vi "Pasco Drive Correcting.vi"(11 "Power":dbl) -> (0 "RightDriveOutput":dbl, 3 "LeftDriveOutput":dbl)   [LabVIEW 2011]
uses:
  Robot Global Data.vi
panel:
  in  "LeftDriveOutput 2":dbl
  in  "RightDriveOutput 2":dbl
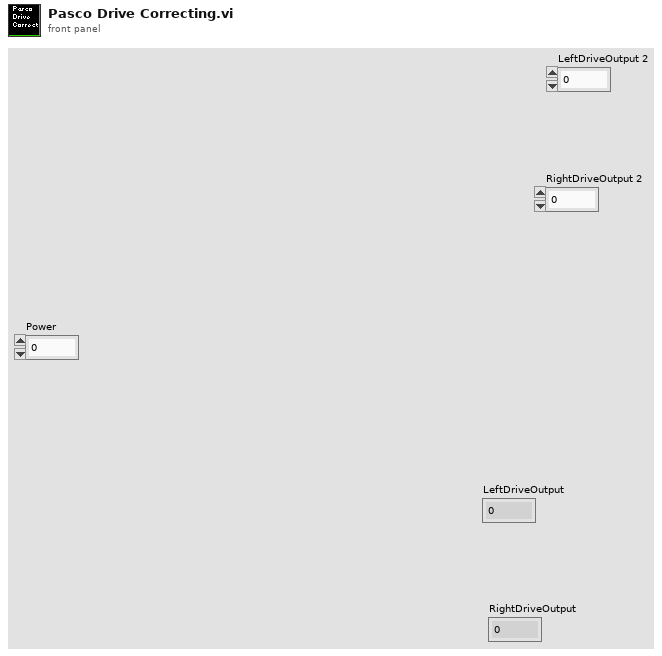
[diagram p1: front panel]
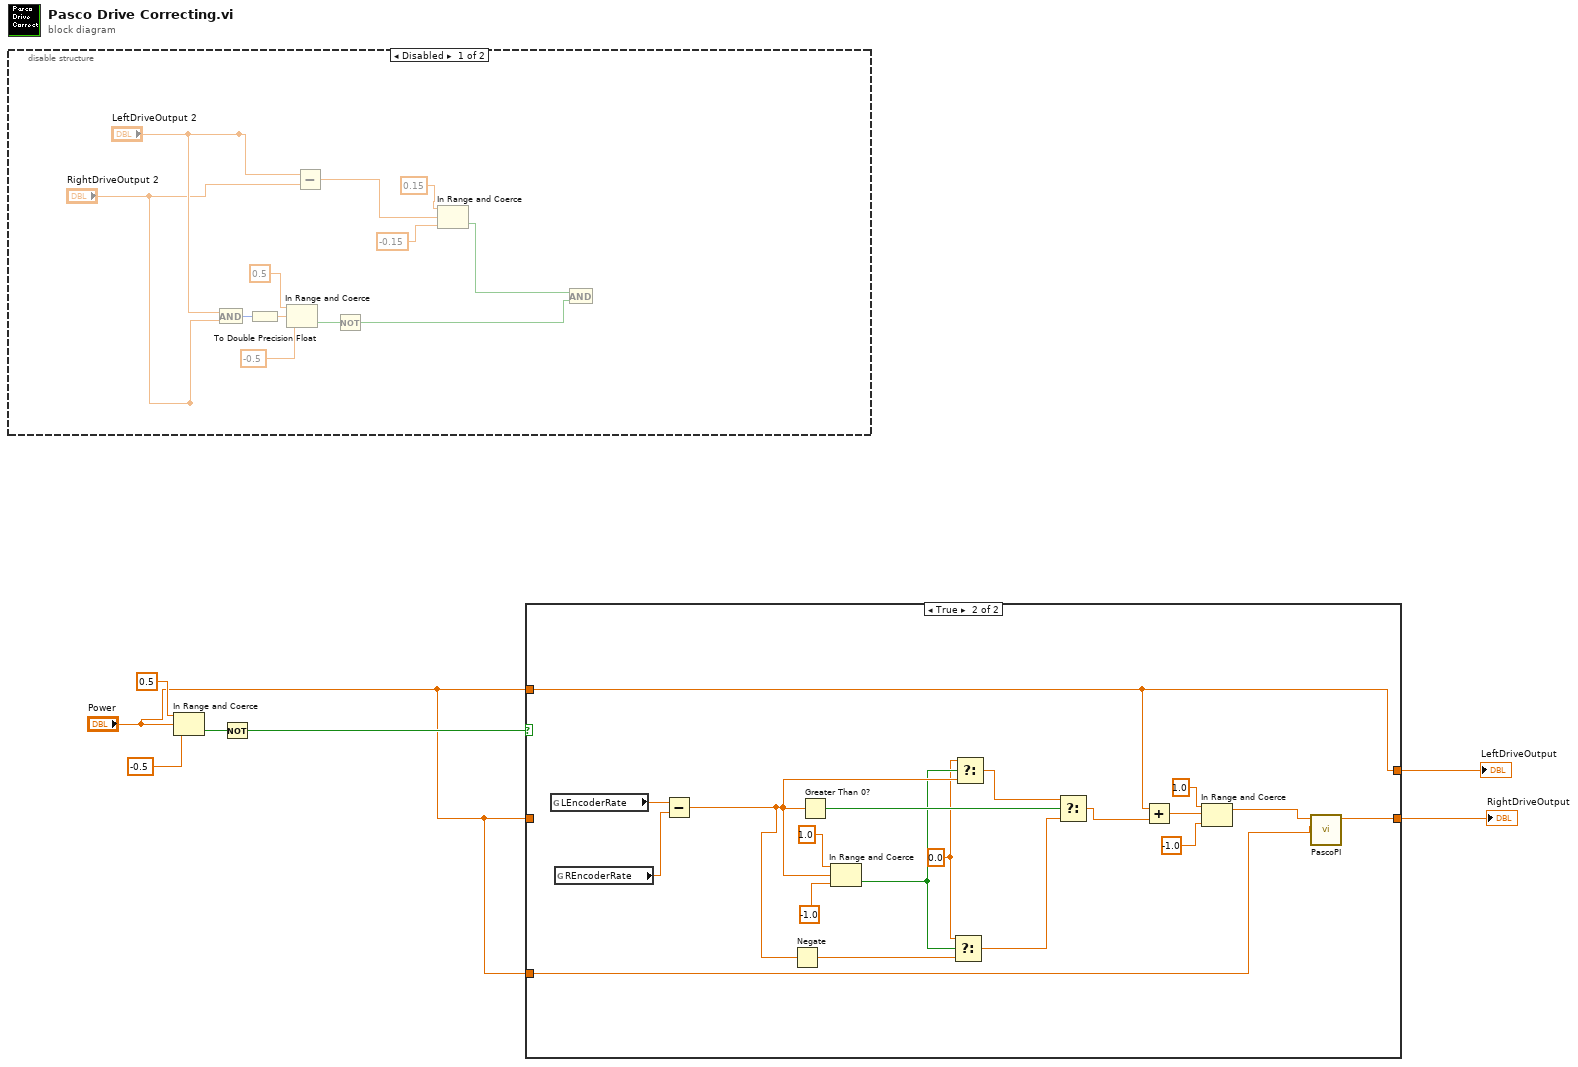
[diagram p0: block diagram]
diagram:
  n1 = disable-structure shown="Disabled" {
    frame Disabled {
      n2 = And(x="LeftDriveOutput 2", y="RightDriveOutput 2") -> (x .and. y?=w12:i32)
      n3 = To Double Precision Float(number=w12) -> (double precision float=w13:dbl)
      n4 = In Range and Coerce(upper limit=0.5, x=w13, lower limit=-0.5) -> (In Range?=w16:bool)  [unwired: 1 out]
      n5 = Subtract(x="LeftDriveOutput 2", y="RightDriveOutput 2") -> (x-y=w9:dbl)
      n6 = Not(x=w16) -> (.not. x?=w17:bool)
      n7 = In Range and Coerce(upper limit=0.15, x=w9, lower limit=-0.15 ("upper limit")) -> (In Range?=w8:bool)  [unwired: 1 out]
      n8 = And(x=w8, y=w17) -> ()  [unwired: 1 out]
    }
    frame Enabled {
    }
  }
  n9 = In Range and Coerce(upper limit=0.5, x="Power", lower limit=-0.5) -> (In Range?=w5:bool)  [unwired: 1 out]
  n10 = Not(x=w5) -> (.not. x?=w2:bool)
  n11 = case shown="True" w2 {
    tunnel: [w21 w24] -> w4
    tunnel: "Power" -> [w21 _]
    tunnel: [w20 w22] -> w3
    tunnel: "Power" -> [w20 w22]
    tunnel: "Power" -> [_ w23]
    frame False {
    }
    frame True {
      w29 = 0.0
      n12 = global read "Robot Global Data.vi" "LEncoderRate"() -> (w40:dbl)
      n13 = global read "Robot Global Data.vi" "REncoderRate"() -> (w39:dbl)
      n14 = Subtract(x=w40, y=w39) -> (x-y=w32:dbl)
      n15 = Negate(x=w32) -> (-x=w33:dbl)
      n16 = Greater Than 0?(x=w32) -> (x > 0?=w38:bool)
      n17 = In Range and Coerce(upper limit=1.0, x=w32, lower limit=-1.0 ("upper limit")) -> (In Range?=w30:bool)  [unwired: 1 out]
      n18 = Select(t=w29, s=w30, f=w33) -> (s? t:f=w34:dbl)
      n19 = Select(t=w29, s=w30, f=w32) -> (s? t:f=w35:dbl)
      n20 = Select(t=w35, s=w38, f=w34) -> (s? t:f=w31:dbl)
      n21 = Add(x=w22, y=w31) -> (x+y=w28:dbl)
      n22 = In Range and Coerce(upper limit=1.0, x=w28, lower limit=-1.0 ("upper limit")) -> (coerced(x)=w25:dbl)  [unwired: 1 out]
      n23 = call "PascoPI.vi"("Feedback"=w23, "Setpoint"=w25) -> ("Motor Output"=w24:dbl)  [unwired: 9 in]
    }
  }
  "LeftDriveOutput" <- w3
  "RightDriveOutput" <- w4
